vi "Helm Check for timeout.vi"(8 "error in (no error)":errorcluster, 10 "Command":enum16{"Steering Command", "Heading Command"}(ring), 11 "RDS Helm Actor in":refnum<class "RDS Helm Actor.lvclass">) -> (0 "error out":errorcluster, 3 "RDS Helm Actor out":refnum<class "RDS Helm Actor.lvclass">)   [LabVIEW 2015, in "RDS Helm Actor.lvlib" / "RDS Helm Actor.lvclass"]
uses:
  RDS Helm Actor.lvclass
  RDS Helm Actor.lvclass/RDS Helm Actor.ctl
  Helm State.ctl
  RDS Helm Actor.lvlib
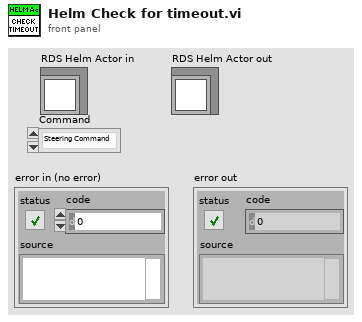
[diagram p1: front panel]
types:
  T1 = typedef "RDS Helm Actor.lvlib/Helm State.ctl" = enum16{"Idle", "Executing Heading Command", "Executing Steering Command"}
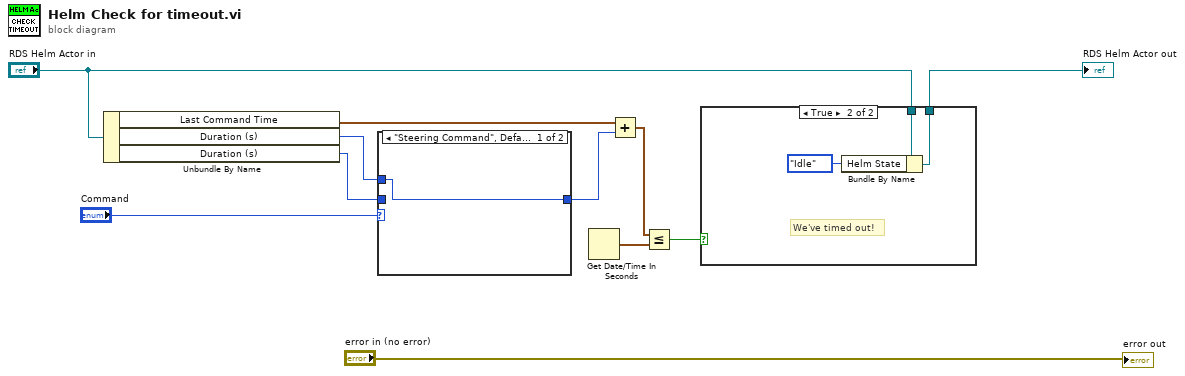
[diagram p0: block diagram]
diagram:
  n1 = Unbundle By Name("RDS Helm Actor in") -> ("Last Command Time"=w6:timestamp, "Duration (s)"=w1:u16, "Duration (s)"=w2:i16)
  n2 = case shown="\"Steering Command\", Default" "Command" {
    tunnel: [w12 w13] -> w3
    tunnel: w2 -> [_ w13]
    tunnel: w1 -> [w12 _]
    frame "Steering Command", Default {
    }
    frame "Heading Command" {
    }
  }
  n3 = Get Date/Time In Seconds() -> (seconds since 1Jan1904=w9:timestamp)
  n4 = Add(x=w6, y=w3) -> (x+y=w8:timestamp)
  n5 = Less Or Equal?(x=w8, y=w9) -> (x <= y?=w7:bool)
  n6 = case shown="True" w7 {
    tunnel: "RDS Helm Actor in" -> [w14 w17]
    tunnel: [w14 w15] -> w11
    frame False {
    }
    frame True {
      # "We've timed out!"
      n7 = Bundle By Name(cluster=w17, "Helm State"=Helm_State."Idle") -> (w15:refnum<class "RDS Helm Actor.lvclass">)
    }
  }
  "RDS Helm Actor out" <- w11
  "error out" <- "error in (no error)"
